vi "ErrorLog_ShowErrorDialog.vi"(7 "Owner (\"\"=All)":string, 8 "error in (no error)":errorcluster, 11 "reference in":refnum<class "ErrorLog.lvclass">) -> (0 "error out":errorcluster, 3 "reference out":refnum<class "ErrorLog.lvclass">)   [LabVIEW 2023, in "ErrorLog.lvclass"]
doc: "Shows Error Dialog"
uses:
  ErrorLog.lvclass
panel:
  in  "pop":bool
  in  "CLR":bool
  out "Errors":string
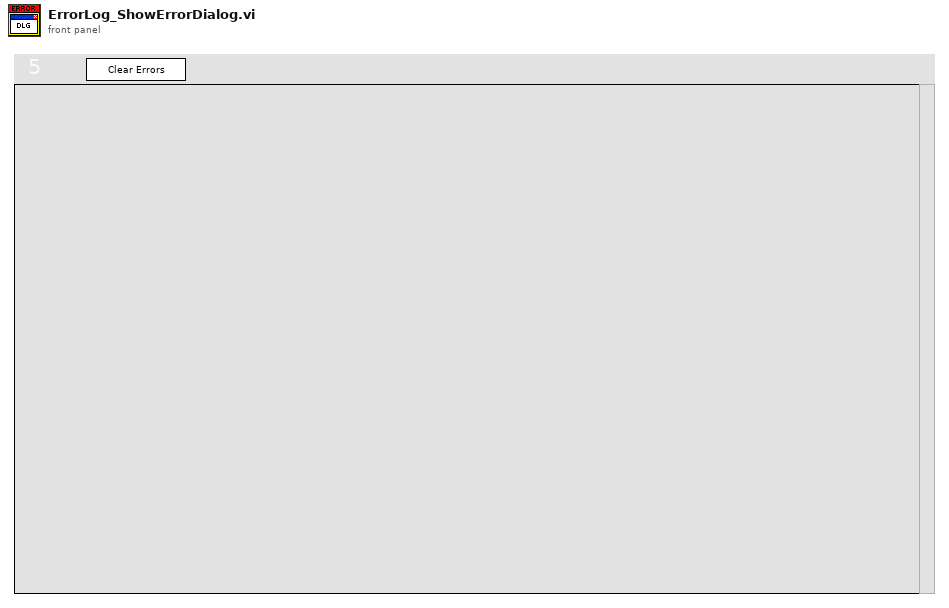
[diagram p1: front panel]
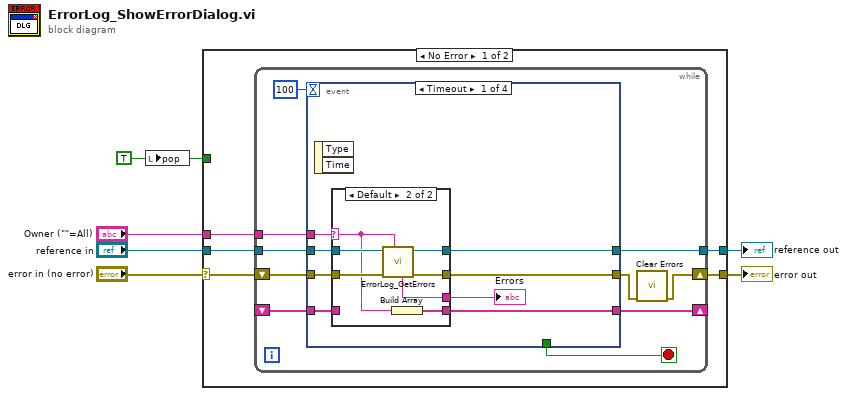
[diagram p0: block diagram]
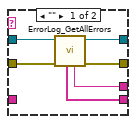
[diagram p2: hidden frame]
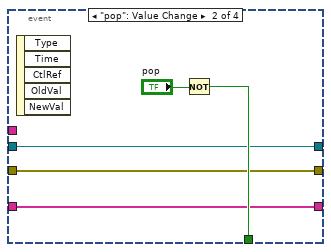
[diagram p3: hidden frame]
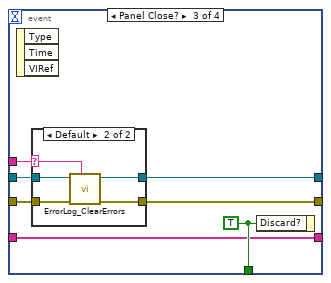
[diagram p4: hidden frame]
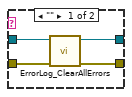
[diagram p5: hidden frame]
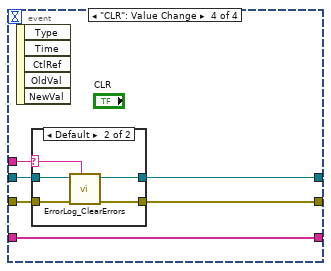
[diagram p6: hidden frame]
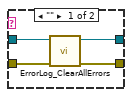
[diagram p7: hidden frame]
diagram:
  w4 = TRUE
  n1 = local write "pop"(w4) -> ()
  n2 = case shown="No Error" "error in (no error)" {
    selector: "error in (no error)" -> [w10 w79]
    tunnel: "reference in" -> [w11 w80]
    tunnel: w4 -> [_ _]
    tunnel: [w9 w80] -> w3
    tunnel: [w8 w79] -> w2
    tunnel: "Owner (\"\"=All)" -> [w7 _]
    frame No Error {
      n3 = while {
        shift-right: [w16] -> w8
        shift-left: w10 -> [w20]
        tunnel: w11 -> [w18]
        tunnel: [w17] -> w9
        tunnel: w7 -> [w14]
        shift-right: [w13] -> _
        shift-left: _ -> [w12]
        stop <- w19 stop-if-true
        n4 = event shown="[0] Timeout" {
          selector: _ -> [_ _ _ _]
          dyn-events: _ -> [_ _ _ _]
          timeout: 100 -> [_ _ _ _]
          tunnel: w20 -> [w29 w45 w52 w67]
          tunnel: [w27 w45 w49 w64] -> w15
          tunnel: [_ w46 w54 _] -> w19
          tunnel: w18 -> [w26 w44 w53 w68]
          tunnel: [w25 w44 w51 w66] -> w17
          tunnel: w14 -> [w24 _ w50 w69]
          tunnel: [w23 w43 w48 w65] -> w13
          tunnel: w12 -> [w22 w43 w48 w65]
          event Timeout {
            n5 = event-data() -> ()  [unwired: 1 in, 2 out]
            n6 = case shown="Default" w24 {
              selector: w24 -> [_ w37]
              tunnel: w29 -> [w34 w42]
              tunnel: [w31 w41] -> w28
              tunnel: [w33 w40] -> w27
              tunnel: w26 -> [w35 w39]
              tunnel: [w32 w38] -> w25
              tunnel: [w30 w36] -> w23
              tunnel: w22 -> [_ _]
              frame "" {
                n7 = call-dynamic "ErrorLog_GetAllErrors.vi"("error in (no error)"=w34, "reference in"=w35) -> ("error out"=w33:errorcluster, "reference out"=w32:refnum<class "ErrorLog.lvclass">, "Errors since last clear"=w31:string, "Error owners since last clear"=w30:string[])  [unwired: 2 in, 4 out]
              }
              frame Default {
                n8 = call-dynamic "ErrorLog_GetErrors.vi"("Owner"=w37, "error in (no error)"=w42, "reference in"=w39) -> ("error out"=w40:errorcluster, "reference out"=w38:refnum<class "ErrorLog.lvclass">, "Errors since last clear"=w41:string)  [unwired: 3 in, 3 out]
                n9 = Build Array(w37) -> (w36:string[])
              }
            }
            "Errors" <- w28
          }
          event "pop": Value Change {
            n10 = event-data() -> ()  [unwired: 1 in, 5 out]
            n11 = Not(x="pop") -> (.not. x?=w46:bool)
          }
          event Panel Close? {
            w54 = TRUE ("Discard?")
            n12 = event-data() -> ()  [unwired: 1 in, 3 out]
            n13 = case shown="Default" w50 {
              selector: w50 -> [_ w59]
              tunnel: w53 -> [w58 w63]
              tunnel: w52 -> [w57 w62]
              tunnel: [w56 w61] -> w49
              tunnel: [w55 w60] -> w51
              frame "" {
                n14 = call-dynamic "ErrorLog_ClearAllErrors.vi"("error in (no error)"=w57, "reference in"=w58) -> ("error out"=w56:errorcluster, "reference out"=w55:refnum<class "ErrorLog.lvclass">)  [unwired: 8 in]
              }
              frame Default {
                n15 = call-dynamic "ErrorLog_ClearErrors.vi"("Owner"=w59, "error in (no error)"=w62, "reference in"=w63) -> ("error out"=w61:errorcluster, "reference out"=w60:refnum<class "ErrorLog.lvclass">)  [unwired: 7 in]
              }
            }
            n16 = event-data("Discard?"=w54) -> ()  [unwired: 1 in, 1 out]
          }
          event "CLR": Value Change {
            n17 = event-data() -> ()  [unwired: 1 in, 5 out]
            n18 = case shown="Default" w69 {
              selector: w69 -> [_ w74]
              tunnel: w68 -> [w73 w78]
              tunnel: w67 -> [w72 w77]
              tunnel: [w71 w76] -> w64
              tunnel: [w70 w75] -> w66
              frame "" {
                n19 = call-dynamic "ErrorLog_ClearAllErrors.vi"("error in (no error)"=w72, "reference in"=w73) -> ("error out"=w71:errorcluster, "reference out"=w70:refnum<class "ErrorLog.lvclass">)  [unwired: 8 in]
              }
              frame Default {
                n20 = call-dynamic "ErrorLog_ClearErrors.vi"("Owner"=w74, "error in (no error)"=w77, "reference in"=w78) -> ("error out"=w76:errorcluster, "reference out"=w75:refnum<class "ErrorLog.lvclass">)  [unwired: 7 in]
              }
            }
          }
        }
        n21 = call <vilib>:"Clear Errors.vi"("error in (no error)"=w15) -> ("error out"=w16:errorcluster)  [unwired: 5 in, 1 out]
      }
    }
    frame Error {
    }
  }
  "error out" <- w2
  "reference out" <- w3
